vi "Set - Time Remaining.vi"(8 "error in (no error)":errorcluster, 10 "Elapsed Time":dbl, 11 "View Model":T1) -> (0 "error out":errorcluster, 3 "View Model":T1)   [LabVIEW 2017]
doc: "Set Elapsed Time actual value to DVR."
uses:
  Controls/View Model.ctl
  Controls/Shared Model.ctl
  Error Handler/Controls/Error Model.ctl
  Error Handler/Controls/Error Data.ctl
  Error Handler/Controls/Error Level.ctl
  Configuration/Controls/Config Model.ctl
  Configuration/Controls/Config Record.ctl
  Configuration/Controls/Config Data.ctl
  Configuration/Controls/Config Command.ctl
  Controller/Controls/Controler Model.ctl
  Views/Entry Console View/Controls/Entry Console - Wash Steps.ctl
  Controller/Controls/Controller - Overhead.ctl
  Controller/Controls/Controller - States.ctl
  Controller/Controls/Controller - Wash Step.ctl
  Views/Vehicle Position View/Controls/Vehicle - Station Enum.ctl
  Controller/Controls/Controller - Event.ctl
  Controller/Controls/Controller - Commands.ctl
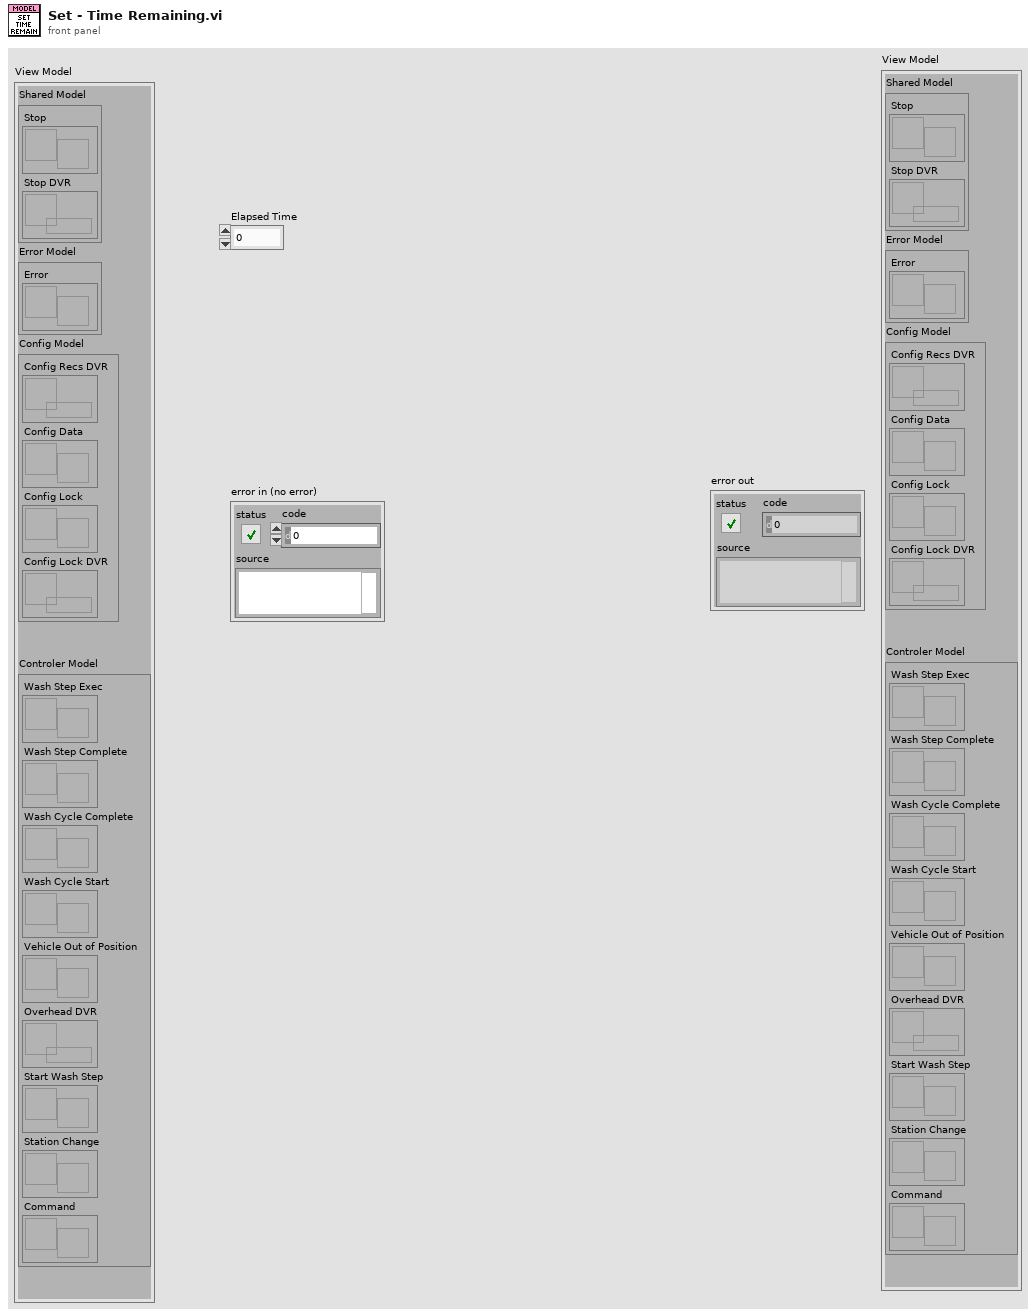
[diagram p1: front panel]
types:
  T1 = typedef "View Model.ctl" = cluster{"Shared Model":T2, "Error Model":T3, "Config Model":T4, "Controler Model":T5}
  T2 = typedef "Shared Model.ctl" = cluster{"Stop":refnum<user-event>, "Stop DVR":refnum<data-value>}
  T3 = typedef "Error Model.ctl" = cluster{"Error":refnum<user-event>}
  T4 = typedef "Config Model.ctl" = cluster{"Config Recs DVR":refnum<data-value>, "Config Data":refnum<user-event>, "Config Lock":refnum<user-event>, "Config Lock DVR":refnum<data-value>}
  T5 = typedef "Controler Model.ctl" = cluster{"Wash Step Exec":refnum<user-event>, "Wash Step Complete":refnum<user-event>, "Wash Cycle Complete":refnum<user-event>, "Wash Cycle Start":refnum<user-event>, "Vehicle Out of Position":refnum<user-event>, "Overhead DVR":refnum<data-value>, "Start Wash Step":refnum<user-event>, "Station Change":refnum<user-event>, "Command":refnum<user-event>}
  T6 = typedef "Controller - Overhead.ctl" = cluster{"Vehicle on Position?":bool, "Step Duration":u32, "Elapsed Time":dbl, "State":T7, "Next State":T7, "Current Wash Step":T8, "Next Wash Step":T8, "Wash Sequence":T8[], "Current Station":T9}
  T7 = typedef "Controller - States.ctl" = enum16{"Initial", "Wait for Start", "Wash Cycle Start", "Wait for Vehicle Position", "Wash Step Start", "Wash Step Execute", "Wash Step Complete", "Wash Cycle Complete", "Wash Exit", "Wash Abort/Terminate"}
  T8 = typedef "Controller - Wash Step.ctl" = enum16{"Under Body Wash", "Bug Remover", "Pre-Soak", "High Pressure Wash", "Low Pressure Wax", "Spot Free Rinse", "Tire Shine Foam", "Air Dry"}
  T9 = typedef "Vehicle - Station Enum.ctl" = enum16{"Entry", "Station1", "Station2", "Station3", "Exit"}
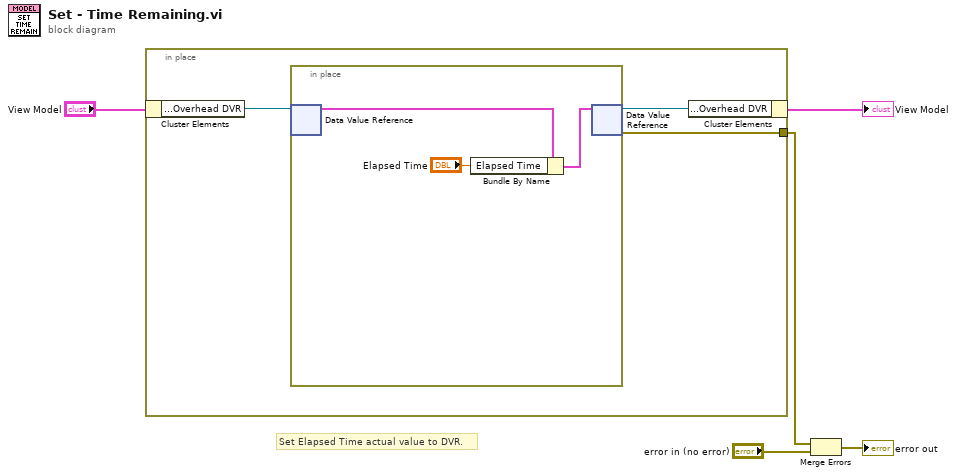
[diagram p0: block diagram]
diagram:
  # "Set Elapsed Time actual value to DVR."
  n1 = in-place {
    in-place-border: [w7] -> w2
    n2 = in-place-cluster #1("View Model") -> ("Controler Model.Overhead DVR"=w6:refnum<data-value>)
    n3 = in-place {
      n4 = in-place-dvr #2(w6) -> (w11:T6)  [unwired: 1 out]
      n5 = Bundle By Name(cluster=w11, "Elapsed Time"="Elapsed Time") -> (w10:T6)
      n6 = in-place-dvr #2(w10) -> (w8:refnum<data-value>, w7:errorcluster)
    }
    n7 = in-place-cluster #1("Controler Model.Overhead DVR"=w8) -> (→"View Model":T1)
  }
  n8 = Merge Errors(w2, "error in (no error)") -> (→"error out":errorcluster)
